vi "Edit-action.vi"(8 "error in (no error)":errorcluster, 11 "Object ref in":T1) -> (0 "error out":errorcluster, 3 "Object ref out":T1)   [LabVIEW 2013, in "PowderDeposition.lvlib" / "PD-Main.lvclass"]
uses:
  PD-Main.lvclass
  Object-reference.ctl
  PD-Main.lvclass/PD-Main.ctl
  Assembly/Motor-assembly.lvclass
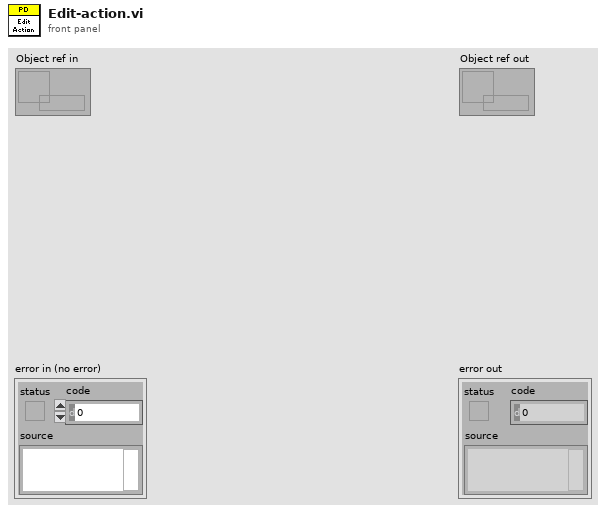
[diagram p1: front panel]
types:
  T1 = typedef "PowderDeposition.lvlib/PD-Main.lvclass/Object-reference.ctl" = refnum<data-value>
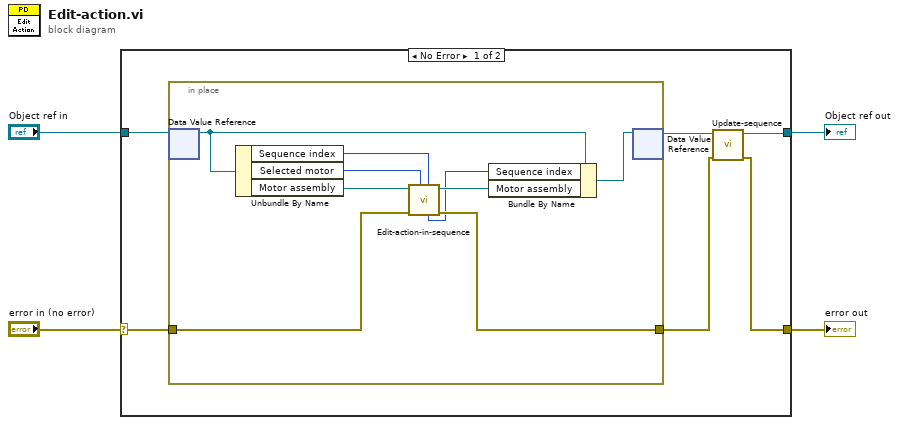
[diagram p0: block diagram]
diagram:
  n1 = case shown="No Error" "error in (no error)" {
    selector: "error in (no error)" -> [w10 w21]
    tunnel: [w5 w21] -> w3
    tunnel: [w7 w20] -> w1
    tunnel: "Object ref in" -> [w9 w20]
    frame No Error {
      n2 = in-place {
        in-place-border: [w19] -> w6
        in-place-border: w10 -> [w18]
        n3 = in-place-dvr #1(w9) -> (w14:refnum<class "PD-Main.lvclass">)  [unwired: 1 out]
        n4 = Unbundle By Name(w14) -> ("Sequence index"=w17:i32, "Selected motor"=w16:i32, "Motor assembly"=w15:refnum<class "Motor-assembly.lvclass">)
        n5 = call "Edit-action-in-sequence.vi"("Sequence index in"=w17, "Motor index"=w16, "error in (no error)"=w18, "Available motors in"=w15) -> ("error out"=w19:errorcluster, "Available motors out"=w12:refnum<class "Motor-assembly.lvclass">, "Sequence index"=w11:i32)  [unwired: 5 in]
        n6 = Bundle By Name(cluster=w14, "Sequence index"=w11, "Motor assembly"=w12) -> (w13:refnum<class "PD-Main.lvclass">)
        n7 = in-place-dvr #1(w13) -> (w8:T1)  [unwired: 1 out]
      }
      n8 = call "Update-sequence.vi"("error in (no error)"=w6, "Object ref in"=w8) -> ("error out"=w5:errorcluster, "Object ref out"=w7:T1)  [unwired: 8 in]
    }
    frame Error {
    }
  }
  "error out" <- w3
  "Object ref out" <- w1
